vi "Configure Trace.vi"(0 "VISA resource name":refnum<visa-resource-name>, 5 "Active Trace (0:A)":i32(ring) items=["A", "B", "C", "D", "E", "F"], 7 "Count (2)":i32=2 min=2 max=9999, 9 "Trace Display Mode (0:Write)":i32(ring) items=["Write", "View", "Blank"], 11 "error in (no error)":errorcluster) -> (4 "VISA resource name out":refnum<visa-resource-name>, 15 "error out":errorcluster)   [LabVIEW 2020, in "Anritsu Signal Analyzer Series.lvlib"]
doc: "Configures the trace settings of the spectrum analyzer."
uses:
  Anritsu Signal Analyzer Series.lvlib
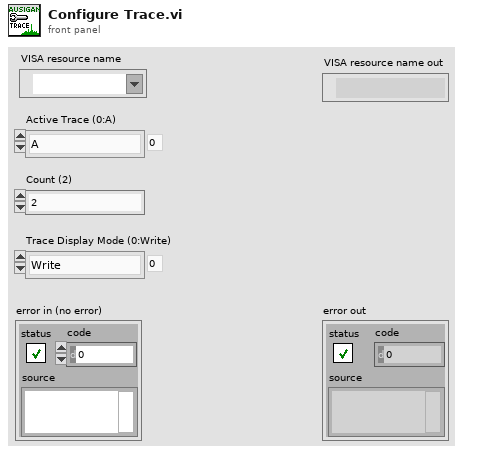
[diagram p1: front panel]
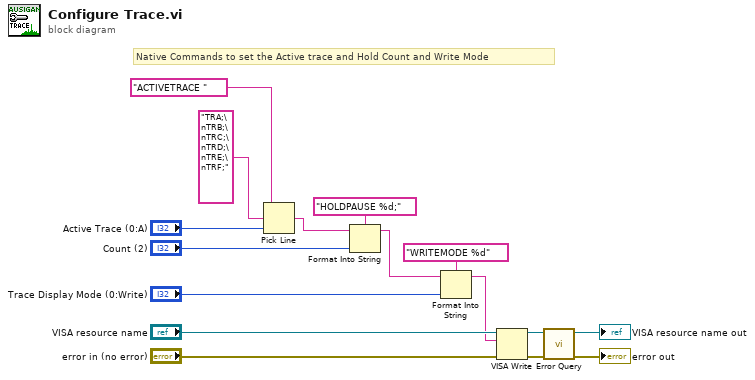
[diagram p0: block diagram]
diagram:
  # "Native Commands to set the Active trace and Hold Count and Write Mode"
  n1 = Pick Line(string ("")="ACTIVETRACE ", multi-line string="TRA;\nTRB;\nTRC;\nTRD;\nTRE;\nTRF;" ("複数行文字列"), line index="Active Trace (0:A)") -> (output string=w1:string)
  n2 = Format Into String(format string="HOLDPAUSE %d;" ("Format String"), initial string=w1, "Count (2)") -> (resulting string=w6:string)  [unwired: 1 in, 1 out]
  n3 = Format Into String(format string="WRITEMODE %d" ("_CommandSet"), initial string=w6, "Trace Display Mode (0:Write)") -> (resulting string=w4:string)  [unwired: 1 in, 1 out]
  n4 = VISA Write(VISA resource name="VISA resource name", write buffer=w4, error in (no error)="error in (no error)") -> (VISA resource name out=w9:refnum<visa-resource-name>, error out=w8:errorcluster)  [unwired: 1 out]
  n5 = call "Error Query.vi"("error in (no error)"=w8, "VISA resource name"=w9) -> ("error out"=→"error out":errorcluster, "VISA resource name out"=→"VISA resource name out":refnum<visa-resource-name>)  [unwired: 6 in, 2 out]
